vi "OAT Scaled Time Domain Window Ex.vi"(2 "window type":u32(ring)=1 items=["None"=0, "Hanning"=1, "Hamming"=2, "Blackman-Harris"=3, "Exact Blackman"=4, "Blackman"=5, "Flat Top"=6, "4 Term B-Harris"=7, "7 Term B-Harris"=8, "Low Sidelobe"=9, "Gaussian"=62], 3 "X":dbl[](array[numeric]) format="%.2f") -> (0 "window constants":cluster{"eq noise BW":dbl, "coherent gain":dbl} {"coherent gain" format="%.2f"; "eq noise BW" format="%.2f"}, 1 "y":dbl[](array[numeric]) format="%.2f")   [LabVIEW 2017]
uses:
  <vilib>/Analysis/4window.llb/windowTd.ctl
  <vilib>/Analysis/0measdsp.llb/Scaled Time Domain Window (DBL).vi
  <vilib>/Analysis/NI_AALPro.lvlib
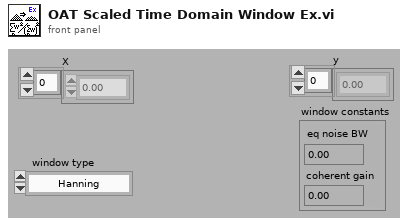
[diagram p1: front panel]
types:
  T1 = typedef "NI_AALPro.lvlib/windowTd.ctl" = u32
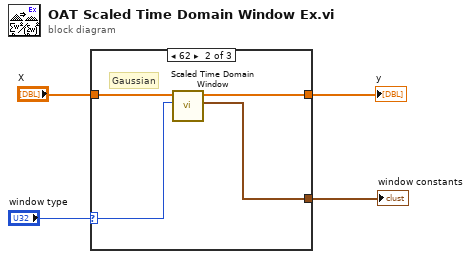
[diagram p0: block diagram]
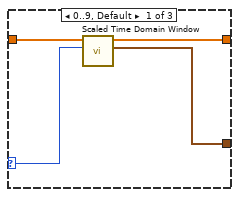
[diagram p2: hidden frame]
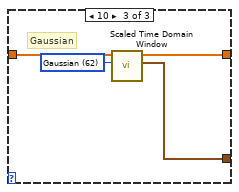
[diagram p3: hidden frame]
diagram:
  n1 = case shown="62" "window type" {
    selector: "window type" -> [w6 w9 _]
    tunnel: "X" -> [w8 w12 w16]
    tunnel: [w7 w11 w15] -> w3
    tunnel: [w5 w10 w14] -> w2
    frame 0..9, Default {
      n2 = call-poly <vilib>:"Scaled Time Domain Window.vi"("window"=w6, "X"=w8) -> ("window properties"=w5:cluster{"eq noise BW":dbl, "coherent gain":dbl}, "Windowed X"=w7:dbl[])  [unwired: 7 in, 1 out]
    }
    frame 62 {
      # "Gaussian"
      n3 = call-poly <vilib>:"Scaled Time Domain Window.vi"("window"=w9, "X"=w12) -> ("window properties"=w10:cluster{"eq noise BW":dbl, "coherent gain":dbl}, "Windowed X"=w11:dbl[])  [unwired: 7 in, 1 out]
    }
    frame 10 {
      w13 = T1 62 items=["Rectangle"=0, "Hanning"=1, "Hamming"=2, "Blackman-Harris"=3, "Exact Blackman"=4, "Blackman"=5, "Flat Top"=6, "4 Term B-Harris "=7, "7 Term B-Harris"=8, "Low Sidelobe"=9, "Blackman Nuttall"=11, "Triangle"=30, "Bartlett-Hanning"=31, "Bohman"=32, "Parzen"=33, "Welch"=34, "Kaiser"=60, "Dolph-Chebyshev"=61, "Gaussian"=62] ("window")
      # "Gaussian"
      n4 = call-poly <vilib>:"Scaled Time Domain Window.vi"("window"=w13, "X"=w16) -> ("window properties"=w14:cluster{"eq noise BW":dbl, "coherent gain":dbl}, "Windowed X"=w15:dbl[])  [unwired: 7 in, 1 out]
    }
  }
  "y" <- w3
  "window constants" <- w2
